vi "PDHydra - GFD Test.vi"(0 "error out 2":errorcluster) -> (3 "Combined Results":string)   [LabVIEW 2022 SP3]
uses:
  <vilib>/Instr/_visa.llb/VISA Flush IO Buffer Mask.ctl
panel:
  out "Unshorted":string
  out "Shorted":string
  out "Unshorted":string
  out "Result (color)":u32(colorbox)
  out "Result (bool)":bool
  in  "OK Button":bool
  in  "bypass":bool
  in  "stop":bool
  out "Inst. Message":string
  out "VISA resource OUT":refnum<visa-resource-name>
  out "error out":errorcluster
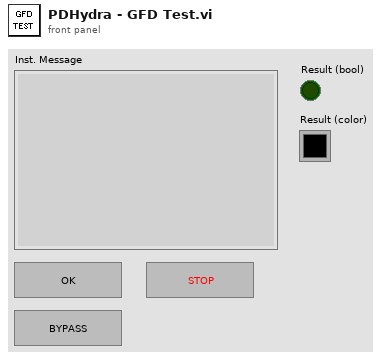
[diagram p1: front panel]
types:
  T1 = typedef "VISA Flush IO Buffer Mask.ctl" = u16
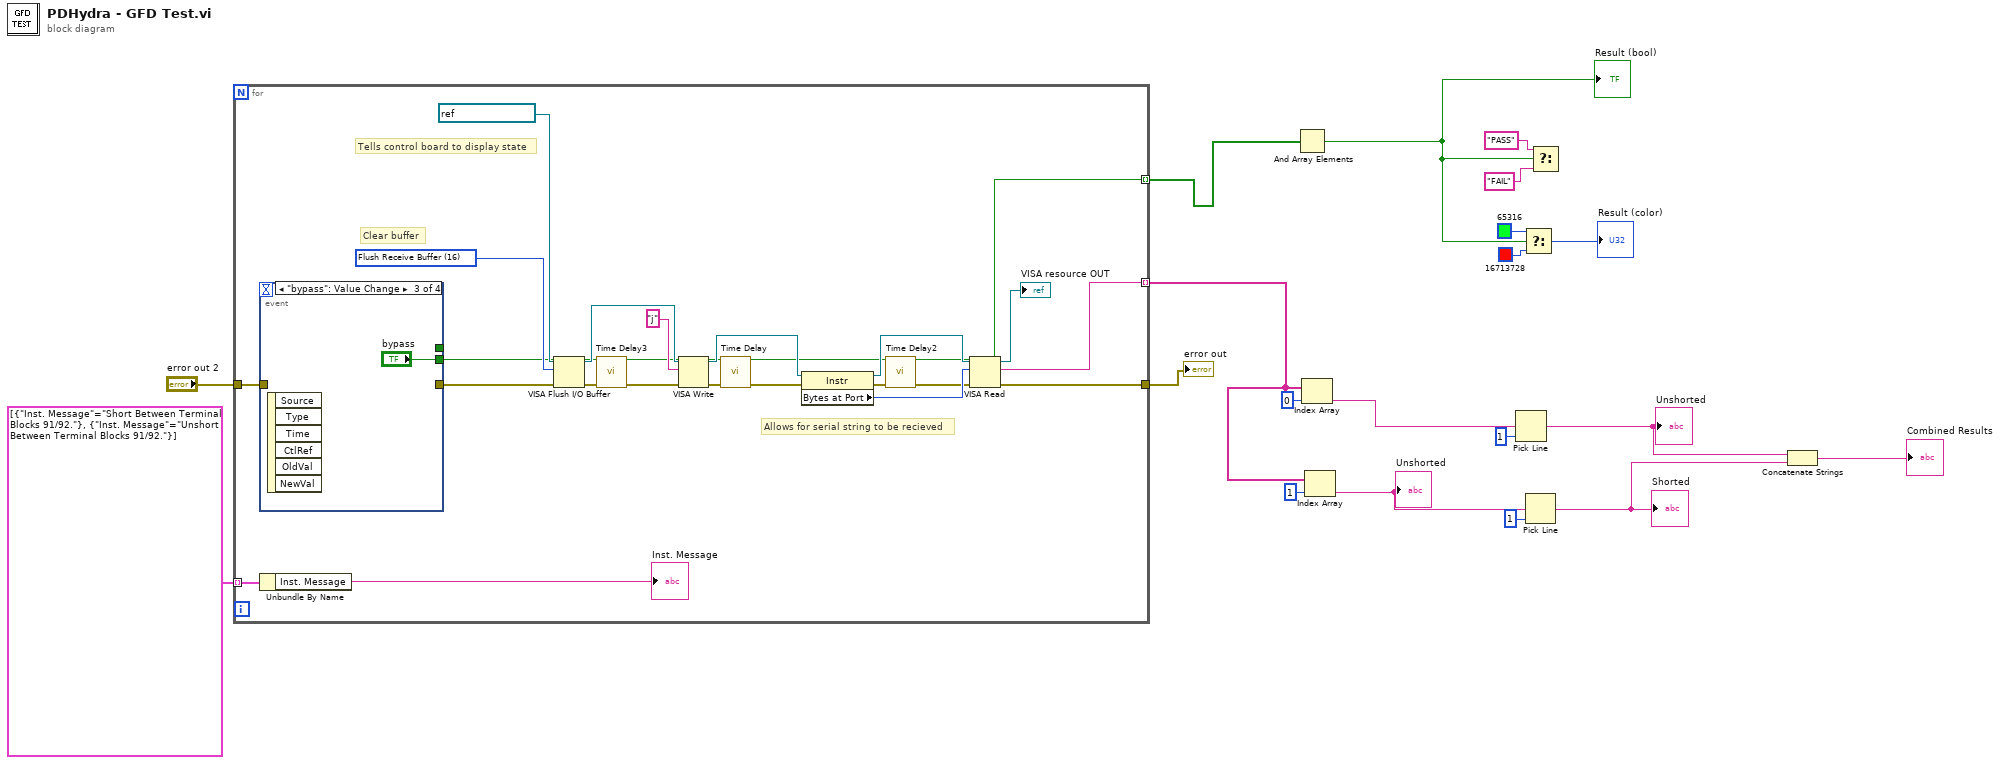
[diagram p0: block diagram]
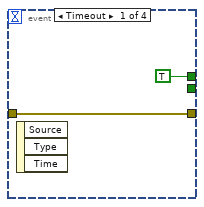
[diagram p2: hidden frame]
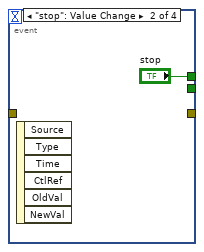
[diagram p3: hidden frame]
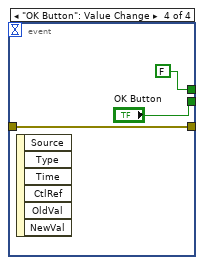
[diagram p4: hidden frame]
diagram:
  n1 = for {
    tunnel: cluster{"Inst. Message":string}[] [{"Inst. Message"="Short Between Terminal Blocks 91/92."}, {"Inst. Message"="Unshort Between Terminal Blocks 91/92."}] -> [w25] mode=indexing
    tunnel: "error out 2" -> [w26]
    tunnel: [w24] -> w12 mode=indexing
    tunnel: [w23] -> w13
    tunnel: [w21] -> w8 mode=indexing
    w38 = T1 16 items=["Flush Receive Buffer"=16, "Write Transmit Buffer to Device"=32, "Flush Receive Buffer (No I/O)"=64, "Flush Transmit Buffer"=128] ("Mask")
    # "Clear buffer"
    # "Allows for serial string to be recieved"
    # "Tells control board to display state"
    n2 = event shown="[2] \"bypass\": Value Change" {
      selector: _ -> [_ _ _ _]
      dyn-events: _ -> [_ _ _ _]
      timeout: _ -> [_ _ _ _]
      tunnel: w26 -> [w43 _ _ w48]
      tunnel: [w43 _ _ w48] -> w27
      tunnel: [TRUE "stop" _ FALSE] -> _
      tunnel: [_ _ "bypass" "OK Button"] -> w24
      event Timeout {
        n3 = event-data() -> ()  [unwired: 1 in, 3 out]
      }
      event "stop": Value Change {
        n4 = event-data() -> ()  [unwired: 1 in, 6 out]
      }
      event "bypass": Value Change {
        n5 = event-data() -> ()  [unwired: 1 in, 6 out]
      }
      event "OK Button": Value Change {
        n6 = event-data() -> ()  [unwired: 1 in, 6 out]
      }
    }
    n7 = Unbundle By Name(w25) -> ("Inst. Message"=→"Inst. Message":string)
    n8 = VISA Flush I/O Buffer(VISA resource name=refnum<visa-resource-name> "ControlBoard", mask (16)=w38, error in (no error)=w27) -> (VISA resource name out=w36:refnum<visa-resource-name>, error out=w29:errorcluster)
    n9 = call "Time Delay3"("error in (no error)"=w29) -> ("error out"=w28:errorcluster)  [unwired: 10 in]
    n10 = VISA Write(VISA resource name=w36, write buffer="j", error in (no error)=w28) -> (VISA resource name out=w34:refnum<visa-resource-name>, error out=w37:errorcluster)  [unwired: 1 out]
    n11 = call "Time Delay"("error in (no error)"=w37) -> ("error out"=w35:errorcluster)  [unwired: 10 in]
    n12 = property class="Instr"(reference=w34, error in=w35) -> (reference out=w40:refnum<visa-resource-name>, error out=w31:errorcluster, "Bytes at Port"=w39:u32)
    n13 = call "Time Delay2"("error in (no error)"=w31) -> ("error out"=w30:errorcluster)  [unwired: 10 in]
    n14 = VISA Read(VISA resource name=w40, byte count=w39, error in (no error)=w30) -> (VISA resource name out=→"VISA resource OUT":refnum<visa-resource-name>, read buffer=w21:string, error out=w23:errorcluster)  [unwired: 1 out]
  }
  "error out" <- w13
  n15 = And Array Elements(Boolean array=w12) -> (logical AND=w11:bool)
  "Result (bool)" <- w11
  n16 = Index Array(array=w8, index=0) -> (element=w5:string)
  n17 = Index Array(array=w8, index=1) -> (element=w6:string)
  "Unshorted" <- w6
  n18 = Pick Line(multi-line string=w5, line index=1) -> (output string=w3:string)  [unwired: 1 in]
  "Unshorted" <- w3
  n19 = Select(t=u32 65316 ("Result (color)"), s=w11, f=u32 16713728 ("Result (color)")) -> (s? t:f=→"Result (color)":u32)
  n20 = Pick Line(multi-line string=w6, line index=1) -> (output string=w2:string)  [unwired: 1 in]
  "Shorted" <- w2
  n21 = Select(t="PASS", s=w11, f="FAIL") -> ()  [unwired: 1 out]
  n22 = Concatenate Strings(w3, w2) -> (→"Combined Results":string)
